vi "GenerateDefaultSVGFile.vi"(8 "error in (no error)":errorcluster) -> (0 "error out":errorcluster, 3 "Path":path)   [LabVIEW 2019]
uses:
  <vilib>/Utility/sysdir.llb/Get System Directory.vi
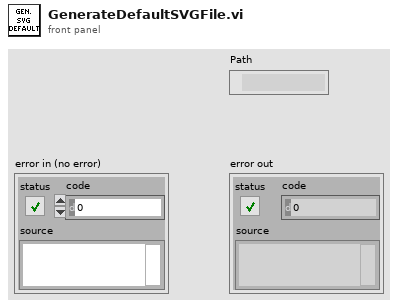
[diagram p1: front panel]
types:
  T1 = enum16{"open", "replace", "create", "open or create", "replace or create", "replace or create with confirmation"}
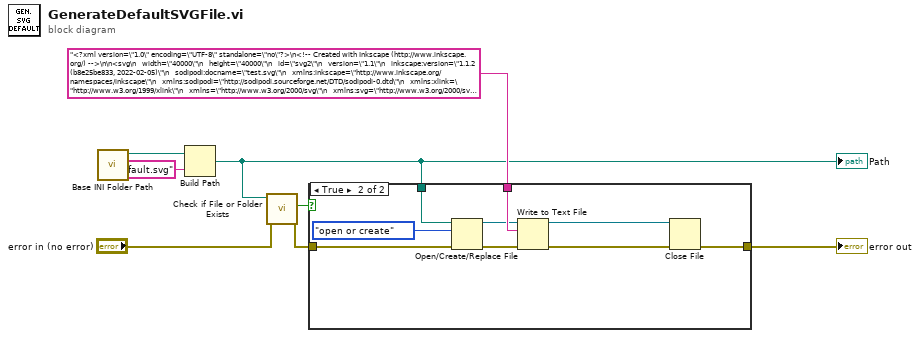
[diagram p0: block diagram]
diagram:
  n1 = call "Base INI Folder Path.vi"() -> ("Base Path"=w8:path)  [unwired: 11 in]
  n2 = Build Path(base path=w8, name or relative path="Default.svg") -> (appended path=w2:path)
  "Path" <- w2
  n3 = call <vilib>:"Check if File or Folder Exists.vi"("error in (no error)"="error in (no error)", "path"=w2) -> ("error out"=w3:errorcluster, "file or folder exists?"=w1:bool)  [unwired: 7 in, 1 out]
  n4 = case shown="True" w1 {
    tunnel: "<?xml version=\"1.0\" encoding=\"UTF-8\" standalone=\"no\"?>\n<!-- Created with Inkscape (http://www.inkscape.org/) -->\n\n<svg\n   width=\"40000\"\n   height=\"40000\"\n   id=\"svg2\"\n   version=\"1.1\"\n   inkscape:version=\"1.1.2 (b8e25be833, 2022-02-05)\"\n   sodipodi:docname=\"test.svg\"\n   xmlns:inkscape=\"http://www.inkscape.org/namespaces/inkscape\"\n   xmlns:sodipodi=\"http://sodipodi.sourceforge.net/DTD/sodipodi-0.dtd\"\n   xmlns:xlink=\"http://www.w3.org/1999/xlink\"\n   xmlns=\"http://www.w3.org/2000/svg\"\n   xmlns:svg=\"http://www.w3.org/2000/svg\"\n   xmlns:rdf=\"http://www.w3.org/1999/02/22-rdf-syntax-ns#\"\n   xmlns:cc=\"http://creativecommons.org/ns#\"\n   xmlns:dc=\"http://purl.org/dc/elements/1.1/\">\n  <defs\n     id=\"defs4\" />\n  <sodipodi:namedview\n     id=\"base\"\n     pagecolor=\"#ffffff\"\n     bordercolor=\"#666666\"\n     borderopacity=\"1.0\"\n     inkscape:pageopacity=\"0.0\"\n     inkscape:pageshadow=\"2\"\n     inkscape:zoom=\"0.014142136\"\n     inkscape:cx=\"17642.314\"\n     inkscape:cy=\"27188.256\"\n     inkscape:document-units=\"px\"\n     inkscape:current-layer=\"svg2\"\n     showgrid=\"false\"\n     inkscape:window-width=\"1920\"\n     inkscape:window-height=\"1001\"\n     inkscape:window-x=\"-9\"\n     inkscape:window-y=\"-9\"\n     inkscape:window-maximized=\"1\"\n     inkscape:showpageshadow=\"false\"\n     inkscape:pagecheckerboard=\"0\" />\n  <metadata\n     id=\"metadata7\">\n    <rdf:RDF>\n      <cc:Work\n         rdf:about=\"\">\n        <dc:format>image/svg+xml</dc:format>\n        <dc:type\n           rdf:resource=\"http://purl.org/dc/dcmitype/StillImage\" />\n        <dc:title />\n      </cc:Work>\n    </rdf:RDF>\n  </metadata>\n  <image\n     id=\"image2993\"\n     xlink:href=\"../../../../../../AFM/surfacepic.jpg\"\n     x=\"0\"\n     y=\"0\"\n     width=\"40000\"\n     height=\"40000\" />\n  <path\n     style=\"fill:#00ff00;fill-opacity:1;stroke:#00fb00;stroke-width:68.42746735;stroke-linecap:butt;stroke-linejoin:miter;stroke-miterlimit:4;stroke-dasharray:none;stroke-opacity:1\"\n     d=\"m 5710.9429,17975.706 44.593,-4593.756 c 1461.0246,971.983 3035.6976,1713.83 4682.3101,2310.003 -1752.8115,344.069 -3431.5235,862.613 -4726.9031,2283.753 z\"\n     id=\"path3768\"\n     inkscape:connector-curvature=\"0\"\n     sodipodi:nodetypes=\"cccc\" />\n  <path\n     style=\"fill:#00ff00;fill-opacity:1;stroke:#00fb00;stroke-width:68.42746735;stroke-linecap:butt;stroke-linejoin:miter;stroke-miterlimit:4;stroke-dasharray:none;stroke-opacity:1\"\n     d=\"m 13400.892,10059.383 4593.756,44.594 c -971.983,1461.024 -1713.83,3035.698 -2310.003,4682.311 -344.069,-1752.812 -862.613,-3431.524 -2283.753,-4726.905 z\"\n     id=\"path3768-1\"\n     inkscape:connector-curvature=\"0\"\n     sodipodi:nodetypes=\"cccc\" />\n  <path\n     style=\"fill:#00ff00;fill-opacity:1;stroke:#00fb00;stroke-width:68.42746735;stroke-linecap:butt;stroke-linejoin:miter;stroke-miterlimit:4;stroke-dasharray:none;stroke-opacity:1\"\n     d=\"m 18739.549,9988.6728 4593.756,44.5932 c -971.983,1461.025 -1713.83,3035.698 -2310.003,4682.311 -344.069,-1752.812 -862.613,-3431.524 -2283.753,-4726.9042 z\"\n     id=\"path3768-9\"\n     inkscape:connector-curvature=\"0\"\n     sodipodi:nodetypes=\"cccc\" />\n  <path\n     style=\"fill:#00ff00;fill-opacity:1;stroke:#00fb00;stroke-width:68.42746735;stroke-linecap:butt;stroke-linejoin:miter;stroke-miterlimit:4;stroke-dasharray:none;stroke-opacity:1\"\n     d=\"m 8100.4383,10879.12 4509.0037,-879.4745 c -658.548,1626.5485 -1068.815,3318.1785 -1321.924,5051.0065 -689.294,-1647.91 -1534.6121,-3188.17 -3187.0797,-4171.532 z\"\n     id=\"path3768-88\"\n     inkscape:connector-curvature=\"0\"\n     sodipodi:nodetypes=\"cccc\" />\n  <path\n     style=\"fill:#00ff00;fill-opacity:1;stroke:#00fb00;stroke-width:68.42746735;stroke-linecap:butt;stroke-linejoin:miter;stroke-miterlimit:4;stroke-dasharray:none;stroke-opacity:1\"\n     d=\"M 29100.623,10575.234 24665.015,9379.4241 c 541.997,1669.0069 831.736,3385.3929 961.8,5131.7729 803.986,-1595.099 1756.002,-3071.794 3473.808,-3935.963 z\"\n     id=\"path3768-88-4\"\n     inkscape:connector-curvature=\"0\"\n     sodipodi:nodetypes=\"cccc\" />\n  <path\n     style=\"fill:#00ff00;fill-opacity:1;stroke:#00fb00;stroke-width:68.42746735;stroke-linecap:butt;stroke-linejoin:miter;stroke-miterlimit:4;stroke-dasharray:none;stroke-opacity:1\"\n     d=\"m 31708.383,17654.207 -44.593,-4593.756 c -1461.024,971.983 -3035.697,1713.83 -4682.31,2310.003 1752.812,344.069 3431.524,862.613 4726.903,2283.753 z\"\n     id=\"path3768-3\"\n     inkscape:connector-curvature=\"0\"\n     sodipodi:nodetypes=\"cccc\" />\n  <path\n     style=\"fill:none;stroke:#00fb00;stroke-width:62.17174911;stroke-linecap:butt;stroke-linejoin:miter;stroke-miterlimit:4;stroke-dasharray:none;stroke-opacity:1\"\n     d=\"m 9075.4469,21348.552 c 0,0 -5.0869,-1278.12 199.2302,-1901.329 280.3951,-855.263 106.6737,-1996.952 1394.6099,-2478.519 1377.731,-515.142 5080.057,-279.059 7627.666,-339.523 1876.994,-44.548 3759.094,-71.272 5635.365,-16.976 1209.741,35.007 2679.222,-238.229 3614.603,220.69 903.916,443.482 984.374,1305.486 1024.612,2003.186 44.859,777.835 -882.304,2274.805 -882.304,2274.805\"\n     id=\"path3856\"\n     inkscape:connector-curvature=\"0\"\n     sodipodi:nodetypes=\"casaaaac\" />\n  <rect\n     style=\"opacity:1;fill:#00ff00;fill-opacity:1;stroke:#000000;stroke-width:0.75590551;stroke-miterlimit:4;stroke-dasharray:none;stroke-opacity:1\"\n     id=\"rect14\"\n     width=\"10288.403\"\n     height=\"5055.8135\"\n     x=\"13547.161\"\n     y=\"20773.98\" />\n  <rect\n     style=\"fill:#00ff00;fill-opacity:1;stroke:#000000;stroke-width:0.693561;stroke-miterlimit:4;stroke-dasharray:none;stroke-opacity:1\"\n     id=\"rect14-8\"\n     width=\"9774.2383\"\n     height=\"4480.123\"\n     x=\"-4974.5957\"\n     y=\"39154.031\"\n     transform=\"matrix(0.87300957,-0.48770308,0.63047396,0.7762104,0,0)\" />\n  <text\n     xml:space=\"preserve\"\n     style=\"font-style:normal;font-weight:normal;font-size:53.3333px;line-height:1.25;font-family:sans-serif;letter-spacing:0px;word-spacing:0px;fill:#000000;fill-opacity:1;stroke:none\"\n     x=\"12020.815\"\n     y=\"20554.562\"\n     id=\"text843\"><tspan\n       sodipodi:role=\"line\"\n       id=\"tspan841\"\n       x=\"12020.815\"\n       y=\"20554.562\">T</tspan></text>\n  <circle\n     style=\"opacity:1;fill:#00ff00;fill-opacity:1;stroke:#000000;stroke-width:1.00157;stroke-miterlimit:4;stroke-dasharray:none;stroke-opacity:1\"\n     id=\"path825\"\n     cx=\"15000\"\n     cy=\"18500\"\n     r=\"100\" />\n  <circle\n     style=\"fill:#00ff00;fill-opacity:1;stroke:#000000;stroke-width:1.00157;stroke-miterlimit:4;stroke-dasharray:none;stroke-opacity:1\"\n     id=\"path825-31\"\n     cx=\"20000\"\n     cy=\"18500\"\n     r=\"100\" />\n  <circle\n     style=\"fill:#00ff00;fill-opacity:1;stroke:#000000;stroke-width:1.00157;stroke-miterlimit:4;stroke-dasharray:none;stroke-opacity:1\"\n     id=\"path825-3\"\n     cx=\"22500\"\n     cy=\"18500\"\n     r=\"100\" />\n  <circle\n     style=\"fill:#00ff00;fill-opacity:1;stroke:#000000;stroke-width:1.00157;stroke-miterlimit:4;stroke-dasharray:none;stroke-opacity:1\"\n     id=\"path825-9\"\n     cx=\"17500\"\n     cy=\"18500\"\n     r=\"100\" />\n  <circle\n     style=\"fill:#00ff00;fill-opacity:1;stroke:#000000;stroke-width:1.00157;stroke-miterlimit:4;stroke-dasharray:none;stroke-opacity:1\"\n     id=\"path825-3-5\"\n     cx=\"25000\"\n     cy=\"18500\"\n     r=\"100\" />\n  <circle\n     style=\"fill:#00ff00;fill-opacity:1;stroke:#000000;stroke-width:1.00157;stroke-miterlimit:4;stroke-dasharray:none;stroke-opacity:1\"\n     id=\"path825-5\"\n     cx=\"13000\"\n     cy=\"20500\"\n     r=\"100\" />\n  <circle\n     style=\"fill:#00ff00;fill-opacity:1;stroke:#000000;stroke-width:1.00157;stroke-miterlimit:4;stroke-dasharray:none;stroke-opacity:1\"\n     id=\"path825-3-4\"\n     cx=\"17000\"\n     cy=\"20500\"\n     r=\"100\" />\n  <circle\n     style=\"fill:#00ff00;fill-opacity:1;stroke:#000000;stroke-width:1.00157;stroke-miterlimit:4;stroke-dasharray:none;stroke-opacity:1\"\n     id=\"path825-9-6\"\n     cx=\"15000\"\n     cy=\"20500\"\n     r=\"100\" />\n  <circle\n     style=\"fill:#00ff00;fill-opacity:1;stroke:#000000;stroke-width:1.00157;stroke-miterlimit:4;stroke-dasharray:none;stroke-opacity:1\"\n     id=\"path825-3-5-2\"\n     cx=\"19000\"\n     cy=\"20500\"\n     r=\"100\" />\n  <path\n     style=\"fill:none;stroke:#00ff00;stroke-width:50;stroke-linecap:butt;stroke-linejoin:miter;stroke-miterlimit:4;stroke-dasharray:none;stroke-opacity:1\"\n     d=\"M 13650,17000 26000,15600\"\n     id=\"path1392\"\n     inkscape:connector-curvature=\"0\" />\n  <path\n     style=\"fill:none;stroke:#00ff00;stroke-width:50;stroke-linecap:butt;stroke-linejoin:miter;stroke-miterlimit:4;stroke-dasharray:none;stroke-opacity:1\"\n     d=\"m 11200,26850 c 1203.007,3334.458 2168.666,2633.989 3250,3900 l 3300,-1750\"\n     id=\"path1394\"\n     inkscape:connector-curvature=\"0\"\n     sodipodi:nodetypes=\"ccc\" />\n</svg>\n" ("text") -> [_ w17]
    tunnel: [w9 w12] -> w5
    tunnel: w3 -> [w9 w11]
    tunnel: w2 -> [_ w10]
    frame False {
    }
    frame True {
      n5 = Open/Create/Replace File(file path (use dialog)=w10, error in=w11, operation (0:open)=T1."open or create") -> (refnum out=w16:refnum<file>, error out=w15:errorcluster)  [unwired: 3 in, 1 out]
      n6 = Write to Text File(file (use dialog)=w16, text=w17, error in=w15) -> (refnum out=w13:refnum<file>, error out=w14:errorcluster)  [unwired: 1 in, 1 out]
      n7 = Close File(refnum=w13, error in=w14) -> (error out=w12:errorcluster)  [unwired: 1 out]
    }
  }
  "error out" <- w5
